vi "Init Tx - Derive Windows Loop Period.vi"(11 "RT Loop Period in":i64) -> (1 "Win Loop Period out":i64, 3 "RT Loop Period out":i64)   [LabVIEW 2016, in "UDP-Custom-Device Engine.lvlib"]
uses:
  UDP-Custom-Device Engine.lvlib
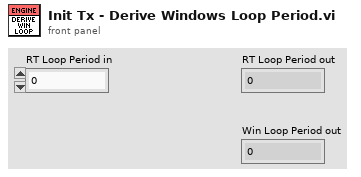
[diagram p1: front panel]
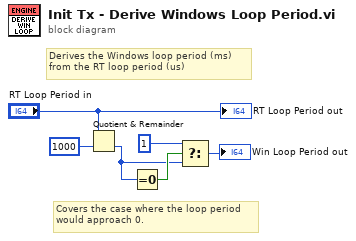
[diagram p0: block diagram]
diagram:
  # "Covers the case where the loop period\nwould approach 0."
  # "Derives the Windows loop period (ms)\nfrom the RT loop period (us)"
  n1 = Quotient & Remainder(x="RT Loop Period in", y=i64 1000 ("x")) -> (floor(x/y)=w3:i64)  [unwired: 1 out]
  n2 = Equal To 0?(x=w3) -> (x = 0?=w4:bool)
  n3 = Select(t=i64 1, s=w4, f=w3) -> (s? t:f=→"Win Loop Period out":i64)
  "RT Loop Period out" <- "RT Loop Period in"
